vi "car feauter using cluster.vi"() -> ()   [LabVIEW 2020]
panel:
  out "output cluster":T1
  in  "form":T1
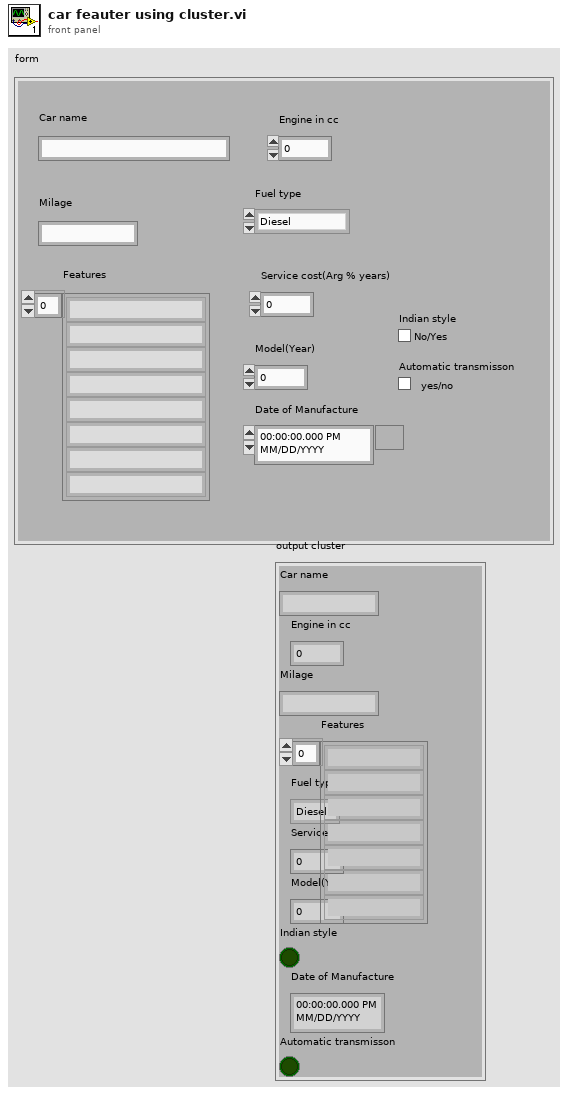
[diagram p1: front panel]
types:
  T1 = cluster{"Car name":string, "Engine in cc":dbl, "Milage":string, "Features":string[], "Fuel type":enum16{"Diesel", "Petrol"}, "Service cost(Arg % years)":dbl, "Model(Year)":dbl, "Indian style":bool, "Date of Manufacture":timestamp, "Automatic transmisson":bool}
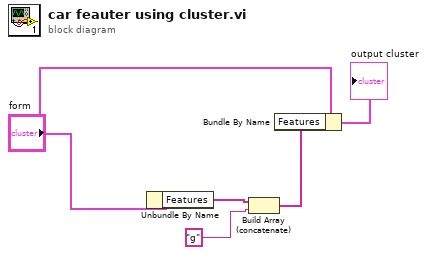
[diagram p0: block diagram]
diagram:
  n1 = Unbundle By Name "Unbundle By Name"("form") -> ("Features"=w4:string[])
  n2 = Build Array (concatenate) "Build Array"(w4, "g") -> (w2:string[])
  n3 = Bundle By Name "Bundle By Name"(cluster="form", "Features"=w2) -> (→"output cluster":T1)
